vi "FilterRecurring.vi"(9 "Error in":errorcluster, 10 "Reset filter?":bool caption="Reset filter? (F)") -> (1 "Error out":errorcluster, 2 "Recurring error filtered?":bool)   [LabVIEW 2017, in "GPError.lvlib"]
doc: "Lets first error of any kind pass through, but clears recurring errors after that no matter their code etc. This is useful in situations where you want to handle the first error only and then suppress consecutive errors, but you don't mind or don't know which error code(s) you'll encounter.\n\nWarnings and 'No error' will always pass through this VI unhindered.\n\n<B>Recurring error filtered?</B> will be True on calls where this VI actually filtered one or more errors.\n\nSet the <B>Reset filter?</B> input temporarily to True to reset this filter, making it revert to its initial state of allowing the first error to pass again.\n\nThis VI supports filtering appended errors.\n\nThis VI is inlined.\n\nSteen Schmidt\nGPower\n18/7 2013"
uses:
  GPError.lvlib
  Append/AppendMulti.vi
panel:
  # "Copyright © 2013\nSteen Schmidt, GPower\nSee enclosed license file for terms and conditions"
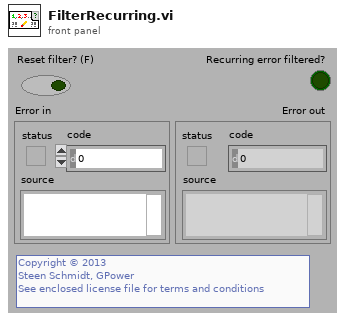
[diagram p1: front panel]
types:
  T1 = typedef "GPError.lvlib/ErrorType.ctl" = enum16{"No Error", "Error", "Warning", "Appended errors", "Appended warnings", "Appended mixed"}
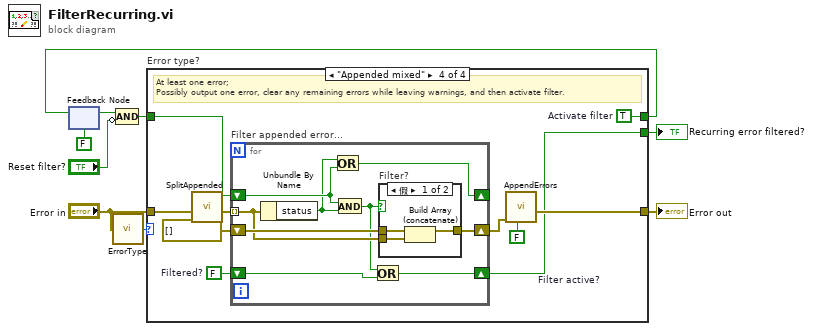
[diagram p0: block diagram]
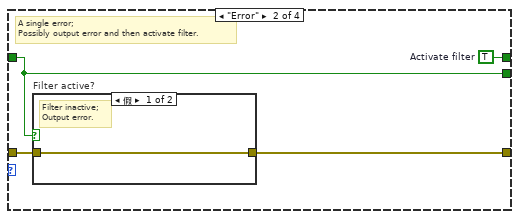
[diagram p3: hidden frame]
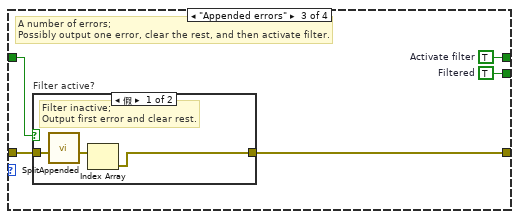
[diagram p5: hidden frame]
diagram:
  n1 = feedback #1 "Filter active?"(FALSE) -> (w8:bool)
  n2 = call "ErrorType.vi"("Error in"="Error in") -> ("Error type"=w6:T1)  [unwired: 4 in]
  n3 = Compound Arithmetic op=AND(w8, invert "Reset filter?") -> (w4:bool)
  n4 = case "Error type?" shown="\"Appended mixed\"" w6 {
    tunnel: "Error in" -> [w11 w15 w21 w34]
    tunnel: w4 -> [w10 w12 w20 w32]
    tunnel: [w11 w14 w19 w29] -> w3
    tunnel: [w10 w13 w18 w28] -> w2
    tunnel: [_ w12 w17 w26] -> w1
    frame "No Error", "Warning", "Appended warnings" {
      # "No error;\nOutput indifferently and leave filter as is."
    }
    frame "Error" {
      w13 = TRUE  # Activate filter
      # "A single error;\nPossibly output error and then activate filter."
      n5 = case "Filter active?" shown="假" w12 {
        tunnel: w15 -> [w16 _]
        tunnel: [w16 _] -> w14
        frame False {
          # "Filter inactive;\nOutput error."
        }
        frame True {
          # "Filter active;\nClear error."
        }
      }
    }
    frame "Appended errors" {
      w17 = TRUE  # Filtered
      w18 = TRUE  # Activate filter
      # "A number of errors;\nPossibly output one error, clear the rest, and then activate filter."
      n6 = case "Filter active?" shown="假" w20 {
        tunnel: w21 -> [w24 _]
        tunnel: [w22 _] -> w19
        frame False {
          # "Filter inactive;\nOutput first error and clear rest."
          n7 = call "SplitAppended.vi"("Appended errors in"=w24) -> ("Errors out"=w23:errorcluster[])  [unwired: 10 in]
          n8 = Index Array(array=w23) -> (element=w22:errorcluster)  [unwired: 1 in]
        }
        frame True {
          # "Filter active;\nClear all errors."
        }
      }
    }
    frame "Appended mixed" {
      w27 = FALSE  # Filtered?
      w28 = TRUE  # Activate filter
      # "At least one error;\nPossibly output one error, clear any remaining errors while leaving warnings, and then activate filter."
      n9 = call "SplitAppended.vi"("Appended errors in"=w34) -> ("Errors out"=w33:errorcluster[])  [unwired: 10 in]
      n10 = for "Filter appended error..." {
        tunnel: w33 -> [w41] mode=indexing
        shift-right: [w38] -> _
        shift-left: w32 -> [w40]
        shift-right: [w42] -> w30
        shift-left: errorcluster[] [] -> [w43]
        shift-right: [w36] -> w26
        shift-left: w27 -> [w35]
        n11 = Unbundle By Name(w41) -> ("status"=w39:bool)
        n12 = Or(x=w39, y=w40) -> (x .or. y?=w38:bool)
        n13 = And(x=w40, y=w39) -> (x .and. y?=w37:bool)
        n14 = Or(x=w37, y=w35) -> (x .or. y?=w36:bool)
        n15 = case "Filter?" shown="假" w37 {
          tunnel: w43 -> [w46 w47]
          tunnel: [w44 w47] -> w42
          tunnel: w41 -> [w45 _]
          frame False {
            n16 = Build Array (concatenate)(w46, w45) -> (w44:errorcluster[])
          }
          frame True {
          }
        }
      }
      n17 = call-poly "AppendErrors.vi"("Only append if new?"=FALSE, "Errors to append"=w30) -> ("Appended errors out"=w29:errorcluster)  [unwired: 9 in]
    }
  }
  "Error out" <- w3
  "Recurring error filtered?" <- w1
  n18 = feedback-in #1(w2) -> ()
